vi "Activity Log Convert to Timestamp.vi"(8 "error in (no error)":errorcluster, 11 "Message Log":string) -> (0 "error out":errorcluster, 2 "Messages":string[](array[string]), 3 "timestamps":timestamp[](array[timestamp]) format="%<%H:%M:%S%3u\n%x>T")   [LabVIEW 2024]
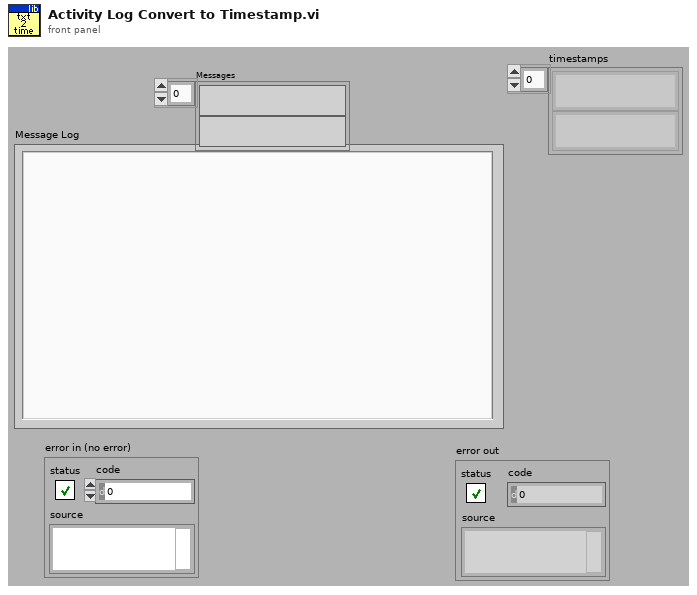
[diagram p1: front panel]
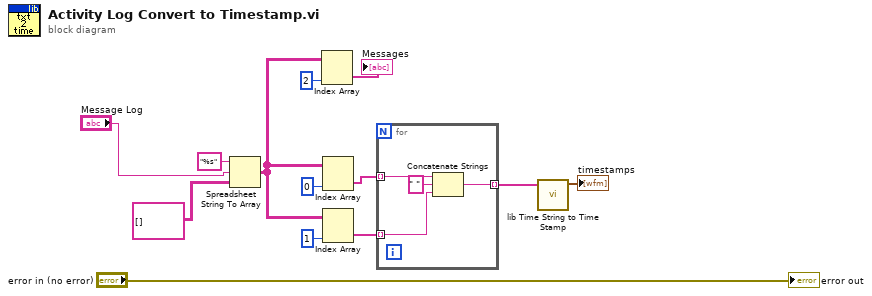
[diagram p0: block diagram]
diagram:
  n1 = Spreadsheet String To Array(format string="%s", spreadsheet string="Message Log", array type (2D Dbl)=string[][] []) -> (array=w4:string[][])  [unwired: 1 in]
  n2 = Index Array(array=w4, index (col)=2 ("disabled index (col)")) -> (element=→"Messages":string[])  [unwired: 1 in]
  n3 = Index Array(array=w4, index (col)=0 ("disabled index (col)")) -> (element=w3:string[])  [unwired: 1 in]
  n4 = Index Array(array=w4, index (col)=1 ("disabled index (col)")) -> (element=w2:string[])  [unwired: 1 in]
  n5 = for {
    tunnel: w3 -> [w17] mode=indexing
    tunnel: w2 -> [w16] mode=indexing
    tunnel: [w14] -> w1 mode=indexing
    n6 = Concatenate Strings(w17, " " ("string"), w16) -> (w14:string)
  }
  n7 = call "lib Time String to Time Stamp.vi"("Array of time strings"=w1) -> ("Array"=→"timestamps":timestamp[])  [unwired: 9 in, 1 out]
  "error out" <- "error in (no error)"
